vi "Data Logging.vi"(0 "VISA resource name":refnum<visa-resource-name>, 5 "Record Number (1)":dbl=1.0 min=1.0 max=1500.0 step=1.0, 7 "Reading Number (1)":dbl=1.0 min=1.0 max=8.0 step=1.0, 11 "error in (no error)":errorcluster) -> (3 "Reading Source":u16(ring) items=["Kelvin", "Celsius", "Sensor Units", "Linear Data"], 4 "VISA resource name out":refnum<visa-resource-name>, 6 "Reading":dbl min=-9999.9 max=9999.9 step=0.0001 format="%.4f", 8 "Date":string, 10 "Time":string, 14 "Relay Status":T1, 15 "error out":errorcluster)   [LabVIEW 2012, in "Lake Shore Cryotronics 218.lvlib"]
doc: "This VI reads a single reading from a logged data record."
uses:
  <instrlib>/Lake Shore Cryotronics 218/Lake Shore Cryotronics 218.lvlib
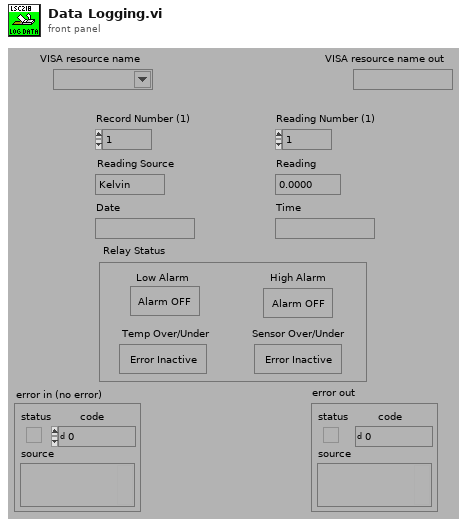
[diagram p1: front panel]
types:
  T1 = cluster{"Low Alarm":bool, "High Alarm":bool, "Temp Over/Under":bool, "Sensor Over/Under":bool}
  T2 = cluster{"Boolean array[0]":bool, "Boolean array[1]":bool, "Boolean array[2]":bool, "Boolean array[3]":bool}
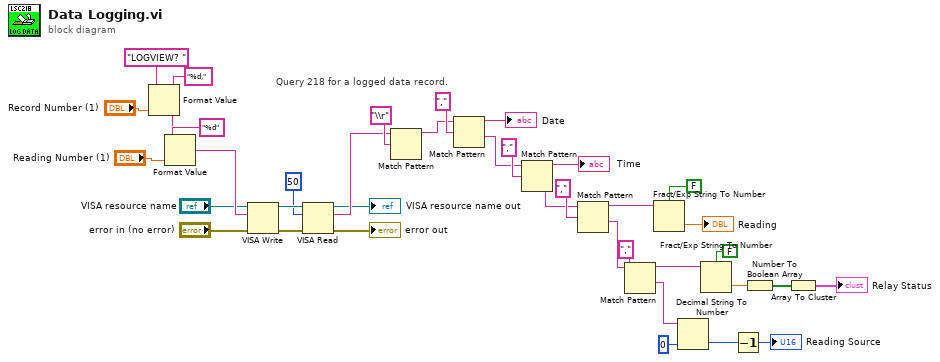
[diagram p0: block diagram]
diagram:
  # "Query 218 for a logged data record."
  n1 = Format Value(string ("")="LOGVIEW? ", format string="%d,", value (0)="Record Number (1)") -> (output string=w29:string)
  n2 = Format Value(string ("")=w29, format string="%d", value (0)="Reading Number (1)") -> (output string=w27:string)
  n3 = VISA Write(VISA resource name="VISA resource name", write buffer=w27, error in (no error)="error in (no error)") -> (VISA resource name out=w34:refnum<visa-resource-name>, error out=w33:errorcluster)  [unwired: 1 out]
  n4 = VISA Read(VISA resource name=w34, byte count=50, error in (no error)=w33) -> (VISA resource name out=→"VISA resource name out":refnum<visa-resource-name>, read buffer=w31:string, error out=→"error out":errorcluster)  [unwired: 1 out]
  n5 = Match Pattern(string=w31, regular expression="\\r") -> (before substring=w22:string)  [unwired: 1 in, 3 out]
  n6 = Match Pattern(string=w22, regular expression=",") -> (before substring=→"Date":string, after substring=w21:string)  [unwired: 1 in, 2 out]
  n7 = Match Pattern(string=w21, regular expression=",") -> (before substring=→"Time":string, after substring=w20:string)  [unwired: 1 in, 2 out]
  n8 = Match Pattern(string=w20, regular expression=",") -> (before substring=w16:string, after substring=w19:string)  [unwired: 1 in, 2 out]
  n9 = Match Pattern(string=w19, regular expression=",") -> (before substring=w14:string, after substring=w10:string)  [unwired: 1 in, 2 out]
  n10 = Fract/Exp String To Number(use system decimal point (T)=FALSE, string=w16) -> (number=→"Reading":dbl)  [unwired: 2 in, 1 out]
  n11 = Decimal String To Number(string=w10, default (0L)=u16 0) -> (number=w9:u16)  [unwired: 1 in, 1 out]
  n12 = Fract/Exp String To Number(use system decimal point (T)=FALSE, string=w14) -> (number=w13:dbl)  [unwired: 2 in, 1 out]
  n13 = Decrement(x=w9) -> (x-1=→"Reading Source":u16)
  n14 = Number To Boolean Array(number=w13) -> (Boolean array=w12:bool[])
  n15 = Array To Cluster(array=w12) -> (cluster=→"Relay Status":T2)
